vi "CLAD1 scratch.vi"() -> ()   [LabVIEW 2013]
panel:
  out "Array - Numeric":dbl[](array[numeric])
  out "Numeric Indicator 2":i32
  out "Numeric Indicator":i32
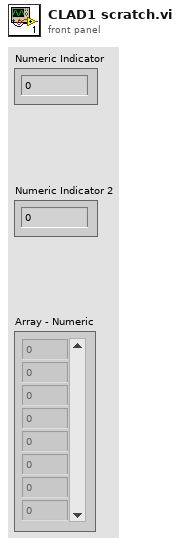
[diagram p1: front panel]
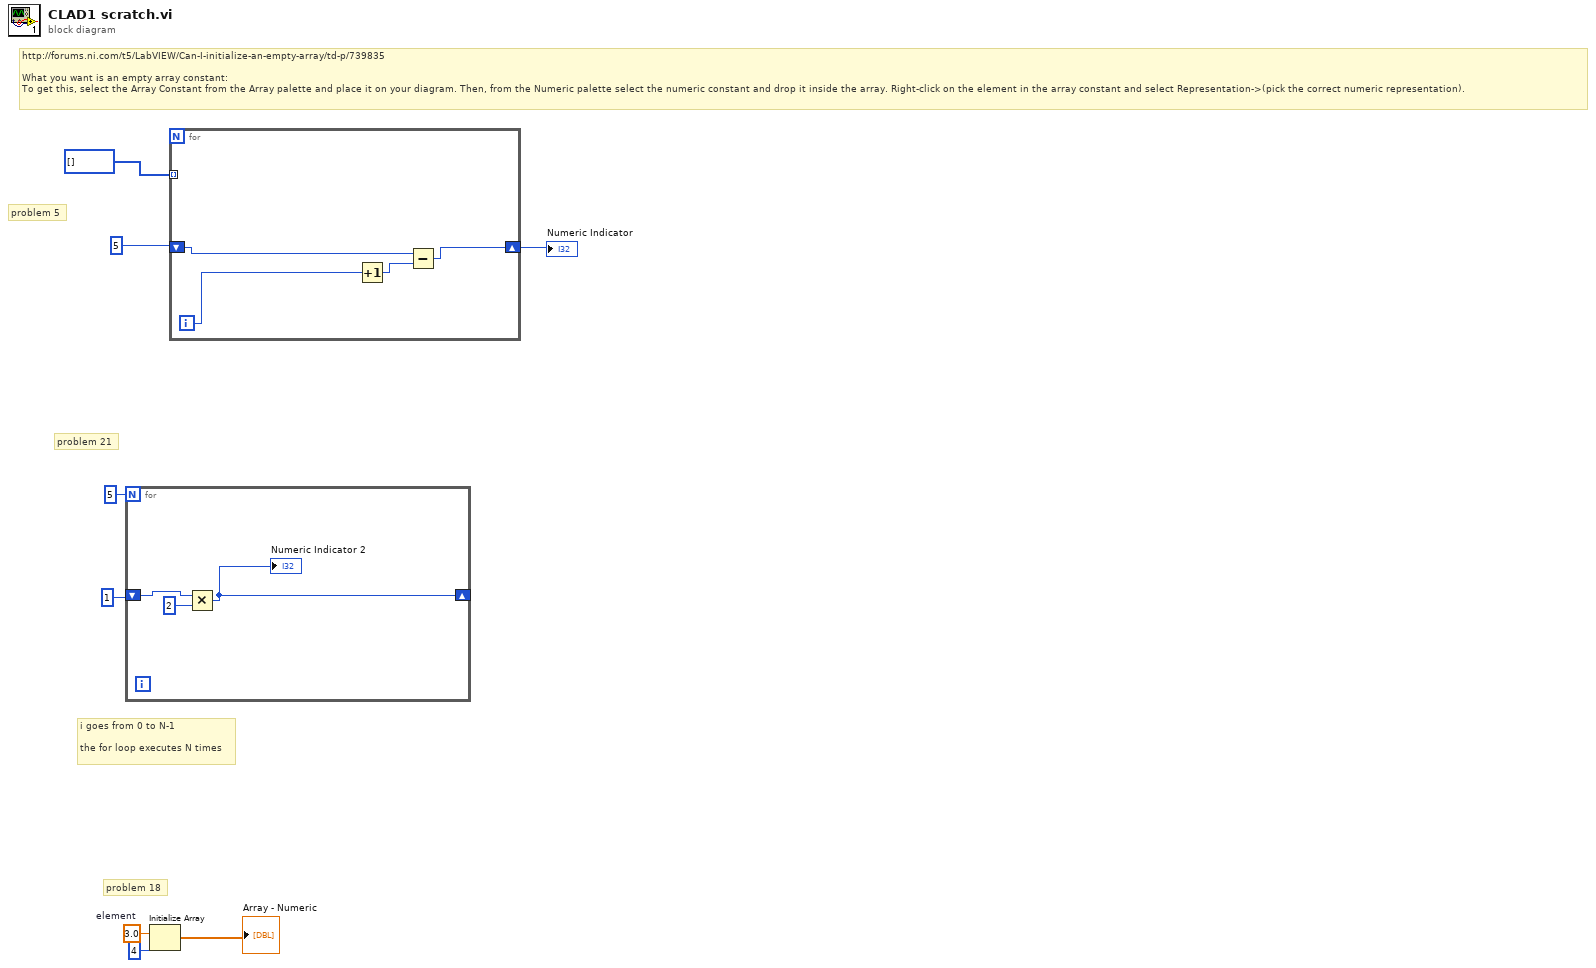
[diagram p0: block diagram]
diagram:
  w3 = 3.0  # element
  # "problem 18"
  # "i goes from 0 to N-1\n\nthe for loop executes N times"
  # "problem 21"
  # "problem 5"
  # "http://forums.ni.com/t5/LabVIEW/Can-I-initialize-an-empty-array/td-p/739835\n\nWhat you want is an empty array constant:\nTo get this, select the Array Constant from the Array palette and place it on your diagram. Then, from the Numeric palette select the numeric constant and drop it inside the array. Right-click on the element in the array constant and select Representation->(pick the correct numeric representation)."
  n1 = for {
    N: 5 -> [_]
    shift-right: [w9] -> _
    shift-left: 1 -> [w10]
    n2 = Multiply(x=w10, y=2) -> (x*y=w9:i32)
    "Numeric Indicator 2" <- w9
  }
  n3 = Initialize Array(w3, 4 ("dimension size")) -> (→"Array - Numeric":dbl[])
  n4 = for {
    tunnel: i32[] [] -> [_] mode=indexing
    shift-right: [w15] -> w6
    shift-left: 5 -> [w14]
    i -> [w13]
    n5 = Increment(x=w13) -> (x+1=w12:i32)
    n6 = Subtract(x=w14, y=w12) -> (x-y=w15:i32)
  }
  "Numeric Indicator" <- w6
